vi "Read Map.vi"(8 "error in":errorcluster, 11 "Ballard ARINC-429 Tx Acyclic execution unit in":refnum<class "Tx Acyclic Labels Execution Unit.lvclass">) -> (0 "error out":errorcluster, 2 "map from values indexes to RT info indexes":T1, 3 "Ballard ARINC-429 Tx Acyclic execution unit out":refnum<class "Tx Acyclic Labels Execution Unit.lvclass">)   [LabVIEW 2020, in "AIM ARINC 429 Engine.lvlib" / "Implementation.lvlib" / "Tx Acyclic Labels Execution Unit.lvclass"]
uses:
  Tx Acyclic Labels Execution Unit.lvclass
  Shared/Map of Values Indexes to Channel and Label Indexes.ctl
  Tx Acyclic Labels Execution Unit.lvclass/Tx Acyclic Labels Execution Unit.ctl
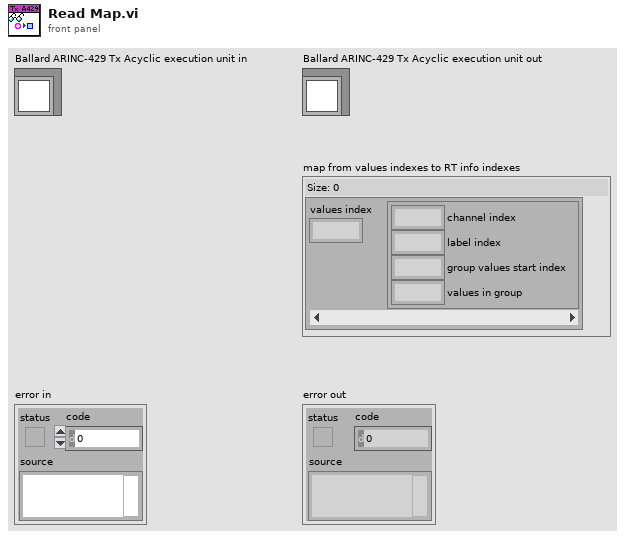
[diagram p1: front panel]
types:
  T1 = typedef "Map of Values Indexes to Channel and Label Indexes.ctl" = map{i32, cluster{"channel index":i32, "label index":i32, "group values start index":i32, "values in group":i32}}
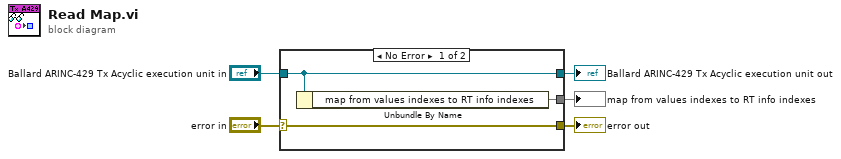
[diagram p0: block diagram]
diagram:
  n1 = case shown="No Error" "error in" {
    selector: "error in" -> [w8 w9]
    tunnel: [w8 w9] -> w4
    tunnel: [w6 w10] -> w2
    tunnel: "Ballard ARINC-429 Tx Acyclic execution unit in" -> [w6 w10]
    tunnel: [w7 _] -> w1
    frame No Error {
      n2 = Unbundle By Name(w6) -> ("map from values indexes to RT info indexes"=w7:T1)
    }
    frame Error {
    }
  }
  "error out" <- w4
  "Ballard ARINC-429 Tx Acyclic execution unit out" <- w2
  "map from values indexes to RT info indexes" <- w1
